vi "Write EndColor.vi"(8 "error in (no error)":errorcluster, 10 "End Color":u32(colorbox), 11 "SliderBG in":refnum<class "SlideBackgroundGradient.lvclass">) -> (0 "error out":errorcluster, 3 "SliderBG out":refnum<class "SlideBackgroundGradient.lvclass">)   [LabVIEW 2023, in "SlideBackgroundGradient.lvclass"]
uses:
  SlideBackgroundGradient.lvclass
  SlideBackgroundGradient.lvclass/SlideBackgroundGradient.ctl
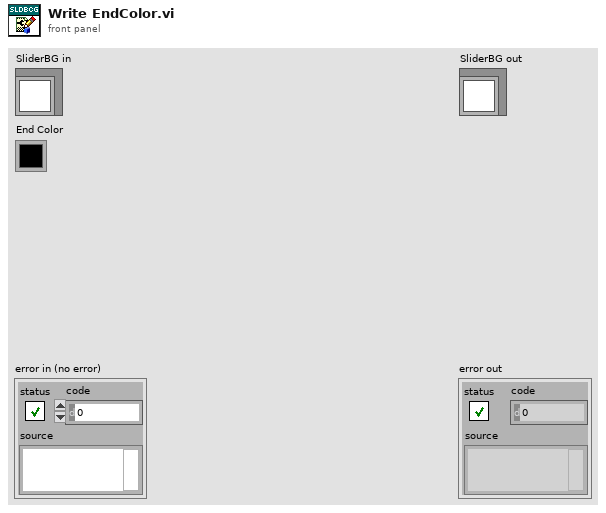
[diagram p1: front panel]
types:
  T1 = typedef "SlideBackgroundGradient.lvclass/State Data.ctl" = cluster{"Start Color":u32, "End Color":u32}
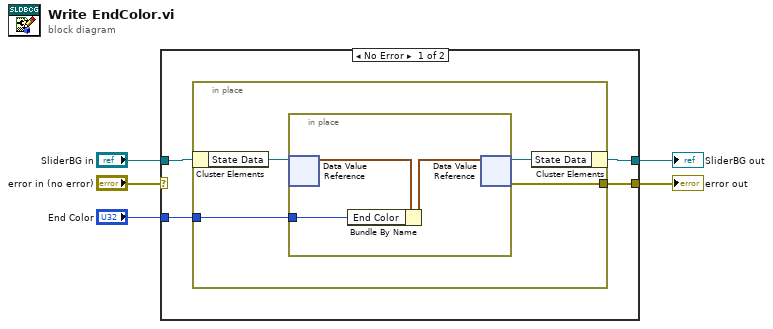
[diagram p0: block diagram]
diagram:
  n1 = case shown="No Error" "error in (no error)" {
    selector: "error in (no error)" -> [_ w18]
    tunnel: [w6 w18] -> w4
    tunnel: [w7 w17] -> w2
    tunnel: "SliderBG in" -> [w9 w17]
    tunnel: "End Color" -> [w8 _]
    frame No Error {
      n2 = in-place {
        in-place-border: w8 -> [w12]
        in-place-border: [w10] -> w6
        n3 = in-place-cluster #1(w9) -> ("State Data"=w13:refnum<data-value>)
        n4 = in-place {
          in-place-border: w12 -> [w15]
          n5 = in-place-dvr #2(w13) -> (w16:T1)  [unwired: 1 out]
          n6 = Bundle By Name(cluster=w16, "End Color"=w15) -> (w14:T1)
          n7 = in-place-dvr #2(w14) -> (w11:refnum<data-value>, w10:errorcluster)
        }
        n8 = in-place-cluster #1("State Data"=w11) -> (w7:refnum<class "SlideBackgroundGradient.lvclass">)
      }
    }
    frame Error {
    }
  }
  "error out" <- w4
  "SliderBG out" <- w2
